vi "test_DL090211FPGA.vi"() -> ()   [LabVIEW 2010, in "FPGAWrapperDL090211Galvo.lvclass"]
uses:
  FPGAWrapperDL090211Galvo.lvclass
  common_typedefs/channels_cluster.ctl
  common_typedefs/gate_parameters_cluster.ctl
  common/classes/ErrorController/ErrorController/ErrorController.lvclass
  common/classes/ErrorController/ErrorController/class_data.vi
panel:
  in  "gate 1 settings":T1
  in  "channel offsets":T2
  out "error controller loaded?":bool=TRUE
  out "pixel dwell time":dbl[unit]
  out "timed out?":bool
  in  "timeout (ms)":i32=500
  out "DAQ loop counter":i32
  out "channel data block":dbl[][](graph)
  in  "number of channels":i32=3
  in  "block size":i32=10000
  out "DL090211FPGAWrapper out":refnum<class "FPGAWrapperDL090211Galvo.lvclass">
  in  "number of pixels":i64=1000000000
  in  "iterations per pixel":i32=250
  in  "run button":bool
  in  "stop":bool
  in  "create button":bool
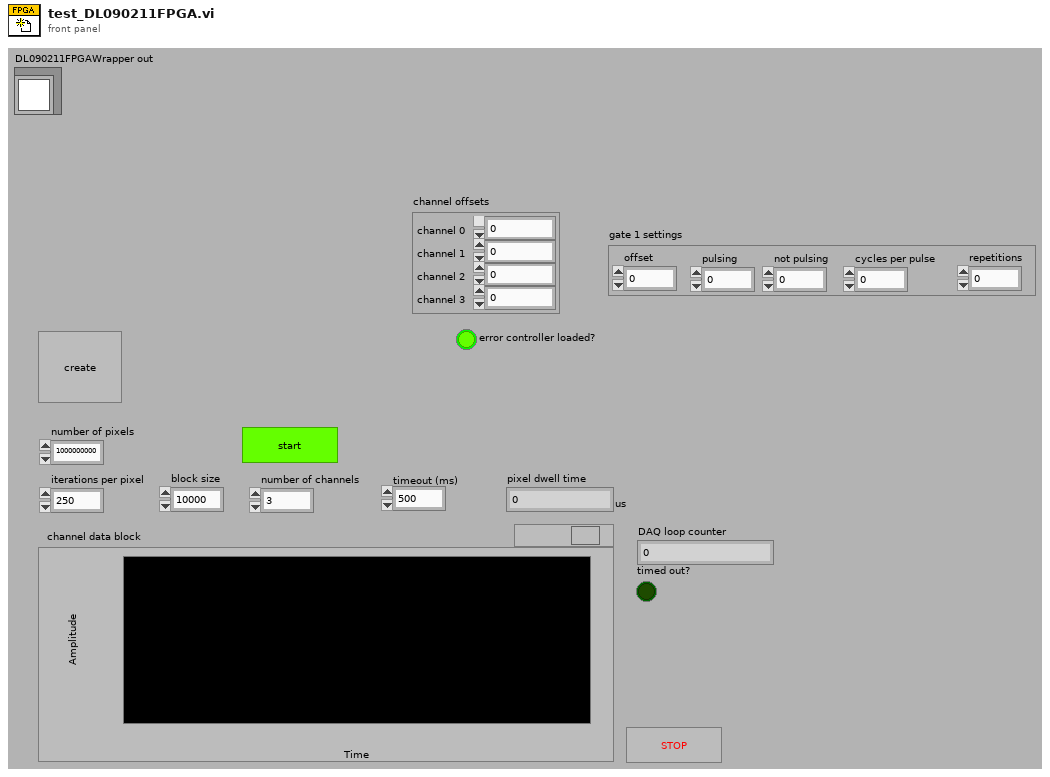
[diagram p1: front panel]
types:
  T1 = typedef "gate_parameters_cluster.ctl" = cluster{"offset":i64, "pulsing":i64, "not pulsing":i64, "cycles per pulse":i64, "repetitions":i64}
  T2 = typedef "channels_cluster.ctl" = cluster{"channel 0":u32, "channel 1":u32, "channel 2":u32, "channel 3":u32}
  T3 = typedef "pixel_raw_data_array.ctl" = dbl[][]
  T4 = typedef "plugin_specification.ctl" = cluster{"class path":string, "configuration":string, "label":string, "settings name":string}
  T5 = typedef "XComponentSpecification.xctl/data.ctl" = cluster{"class path":string, "configuration":string, "label":string, "settings name":string}
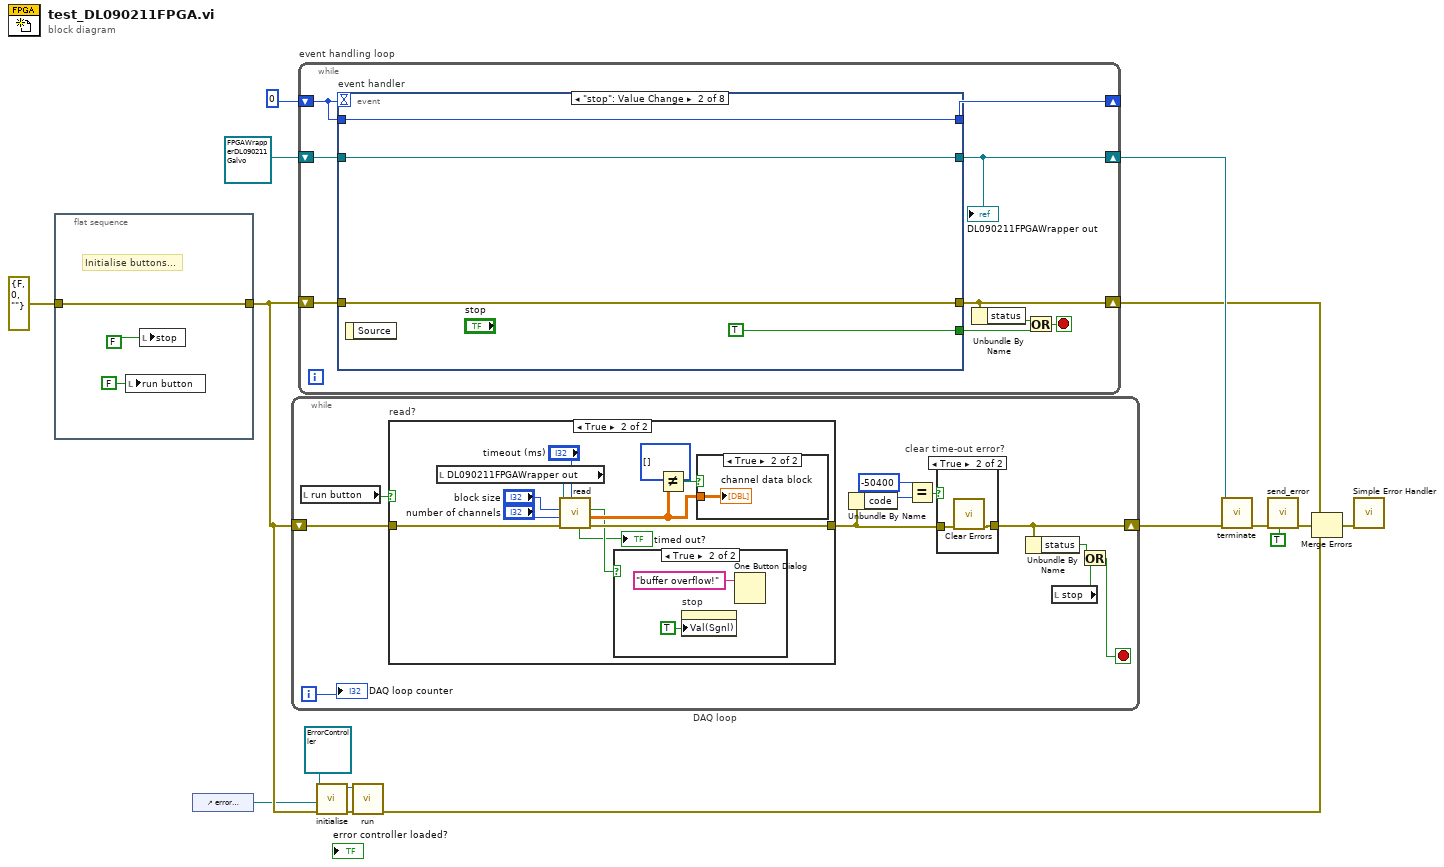
[diagram p0: block diagram]
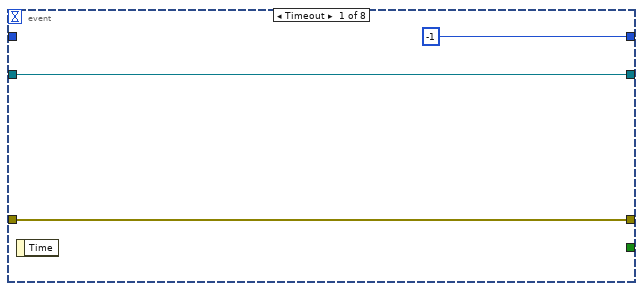
[diagram p6: hidden frame]
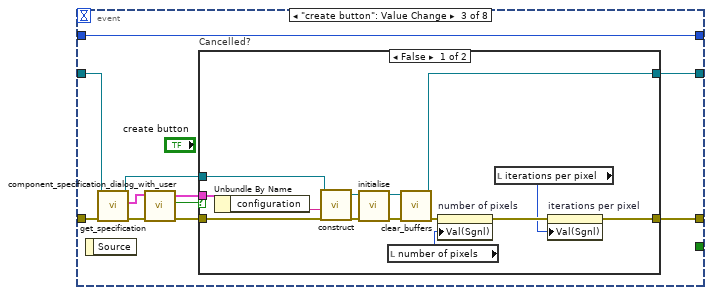
[diagram p7: hidden frame]
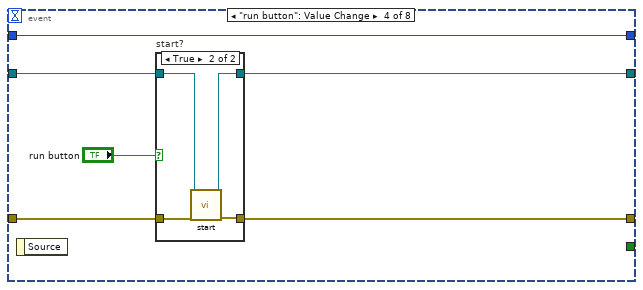
[diagram p9: hidden frame]
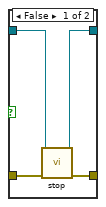
[diagram p10: hidden frame]
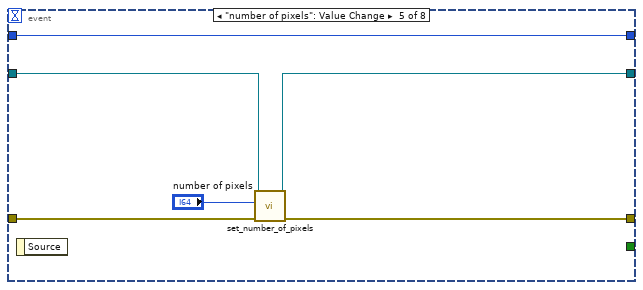
[diagram p11: hidden frame]
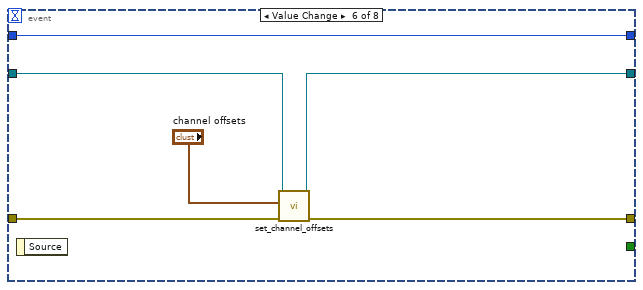
[diagram p12: hidden frame]
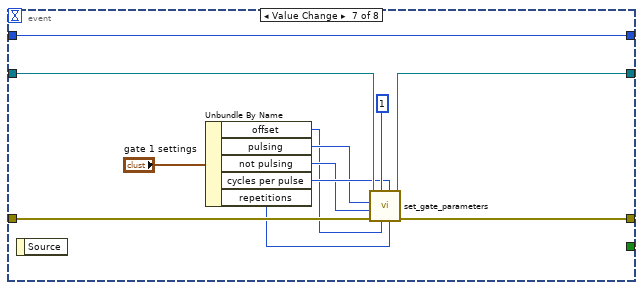
[diagram p13: hidden frame]
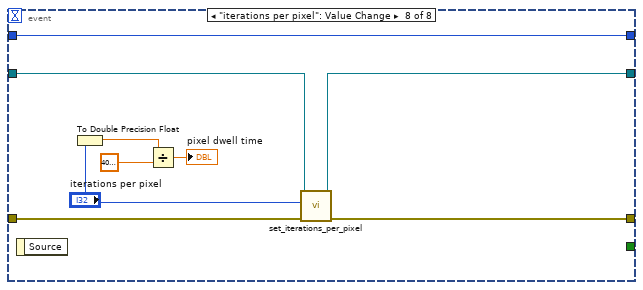
[diagram p14: hidden frame]
diagram:
  n1 = flat-sequence {
    tunnel: errorcluster {"status"=FALSE, "code"=0, "source"=""} ("error in (no error)") -> [w19]
    tunnel: [w19] -> w6
    frame #0 {
      # "Initialise buttons..."
      n2 = local write "run button"(FALSE ("run button")) -> ()
      n3 = local write "stop"(FALSE) -> ()
    }
  }
  n4 = control-ref of="error controller loaded?"() -> (w1:refnum<vi>)
  n5 = while "DAQ loop" {
    shift-right: [w24] -> w13
    shift-left: w6 -> [w30]
    i -> [w20]
    stop <- w21 stop-if-true
    n6 = local read "run button"() -> (w29:bool)
    n7 = case "read?" shown="True" w29 {
      tunnel: w30 -> [w34 w45]
      tunnel: [w34 w44] -> w26
      frame False {
      }
      frame True {
        n8 = local read "DL090211FPGAWrapper out"() -> (w43:refnum<class "FPGAWrapperDL090211Galvo.lvclass">)
        n9 = call-dynamic "read.vi"("timeout (ms)"="timeout (ms)", "error in (no error)"=w45, "number of channels"="number of channels", "block size"="block size", "FPGAWrapperDL090211Galvo in"=w43) -> ("error out"=w44:errorcluster, "channels raw data block"=w39:T3, "FIFO full?"=w37:bool, "timed out?"=→"timed out?":bool)  [unwired: 3 out]
        n10 = case shown="True" w37 {
          frame False {
          }
          frame True {
            n11 = property on="stop" class="Bool (strict)"("Val(Sgnl)"=TRUE) -> ()  [unwired: 2 in, 2 out]
            n12 = One Button Dialog(message="buffer overflow!") -> ()  [unwired: 1 in, 1 out]
          }
        }
        n13 = Not Equal?(x=i32[][] [], y=w39) -> (x != y?=w40:bool)
        n14 = case shown="True" w40 {
          tunnel: w39 -> [_ w48]
          frame False {
          }
          frame True {
            "channel data block" <- w48
          }
        }
      }
    }
    n15 = Unbundle By Name(w26) -> ("code"=w28:i32)
    n16 = Equal?(x=-50400, y=w28) -> (x = y?=w25:bool)
    n17 = case "clear time-out error?" shown="True" w25 {
      tunnel: w26 -> [w31 w33]
      tunnel: [w31 w32] -> w24
      frame False {
      }
      frame True {
        n18 = call <vilib>:"Clear Errors.vi"("error in (no error)"=w33) -> ("error out"=w32:errorcluster)  [unwired: 6 out]
      }
    }
    n19 = Unbundle By Name(w24) -> ("status"=w23:bool)
    n20 = local read "stop"() -> (w22:bool)
    n21 = Or(x=w23, y=w22) -> (x .or. y?=w21:bool)
    "DAQ loop counter" <- w20
  }
  n22 = while "event handling loop" {
    shift-right: [w52] -> w11
    shift-left: w6 -> [w57]
    shift-right: [w55] -> _
    shift-left: 0 -> [w56]
    shift-right: [w53] -> w12
    shift-left: refnum<class "FPGAWrapperDL090211Galvo.lvclass"> refnum ("DL090211FPGAWrapper.lvclass") -> [w54]
    stop <- w49 stop-if-true
    n23 = event "event handler" shown="[1] \"stop\": Value Change" {
      selector: _ -> [_ _ _ _ _ _ _ _]
      dyn-events: _ -> [_ _ _ _ _ _ _ _]
      timeout: w56 -> [_ _ _ _ _ _ _ _]
      tunnel: [w58 w61 w74 w93 w109 w115 w127 w136] -> w52
      tunnel: w57 -> [w58 w61 w71 w96 w110 w116 w128 w137]
      tunnel: w56 -> [_ w64 w75 w97 w111 w117 w129 w138]
      tunnel: [-1 w64 w75 w97 w111 w117 w129 w138] -> w55
      tunnel: [_ TRUE _ _ _ _ _ _] -> w50
      tunnel: [w59 w62 w66 w94 w107 w112 w125 w134] -> w53
      tunnel: w54 -> [w59 w62 w69 w95 w108 w113 w126 w135]
      event Timeout {
        n24 = event-data() -> ()  [unwired: 2 out]
      }
      event "stop": Value Change {
        n25 = event-data() -> ()  [unwired: 2 out]
      }
      event "create button": Value Change {
        n26 = event-data() -> ()  [unwired: 2 out]
        n27 = call-dynamic "get_specification.vi"("error in (no error)"=w71, "GenericPlugin in"=w69) -> ("error out"=w70:errorcluster, "component specification"=w67:T4, "GenericPlugin out"=w68:refnum<class "FPGAWrapperDL090211Galvo.lvclass">)  [unwired: 6 in, 1 out]
        n28 = call "component_specification_dialog_with_user.vi"("error in (no error)"=w70, "component specification in"=w67) -> ("error out"=w73:errorcluster, "cancelled?"=w65:bool, "component specification out"=w72:T5)  [unwired: 7 in]
        n29 = case "Cancelled?" shown="False" w65 {
          tunnel: [w86 w91] -> w74
          tunnel: w73 -> [w80 w91]
          tunnel: w72 -> [w79 _]
          tunnel: w68 -> [w77 w90]
          tunnel: [w76 w90] -> w66
          frame False {
            n30 = Unbundle By Name(w79) -> ("configuration"=w78:string)
            n31 = call-dynamic "construct.vi"("error in (no error)"=w80, "configuration name"=w78, "GenericPlugin in"=w77) -> ("error out"=w82:errorcluster, "GenericPlugin out"=w81:refnum<class "FPGAWrapperDL090211Galvo.lvclass">)  [unwired: 7 in]
            n32 = call-dynamic "initialise.vi"("error in (no error)"=w82, "GenericPlugin in"=w81) -> ("error out"=w85:errorcluster, "GenericPlugin out"=w83:refnum<class "FPGAWrapperDL090211Galvo.lvclass">)  [unwired: 1 in, 7 out]
            n33 = local read "number of pixels"() -> (w87:i64)
            n34 = call-dynamic "clear_buffers.vi"("error in (no error)"=w85, "FPGAWrapperDL090211Galvo in"=w83) -> ("error out"=w84:errorcluster, "FPGAWrapperDL090211Galvo out"=w76:refnum<class "FPGAWrapperDL090211Galvo.lvclass">)  [unwired: 8 in]
            n35 = property on="number of pixels" class="DigNum (strict)"(error in=w84, "Val(Sgnl)"=w87) -> (error out=w89:errorcluster)  [unwired: 1 in, 1 out]
            n36 = local read "iterations per pixel"() -> (w88:i32)
            n37 = property on="iterations per pixel" class="DigNum (strict)"(error in=w89, "Val(Sgnl)"=w88) -> (error out=w86:errorcluster)  [unwired: 1 in, 1 out]
          }
          frame True {
          }
        }
      }
      event "run button": Value Change {
        n38 = event-data() -> ()  [unwired: 2 out]
        n39 = case "start?" shown="True" "run button" {
          tunnel: w96 -> [w101 w105]
          tunnel: w95 -> [w99 w104]
          tunnel: [w98 w103] -> w94
          tunnel: [w100 w102] -> w93
          frame False {
            n40 = call-dynamic "stop.vi"("error in (no error)"=w101, "FPGAWrapperDL090211Galvo in"=w99) -> ("error out"=w100:errorcluster, "FPGAWrapperDL090211Galvo out"=w98:refnum<class "FPGAWrapperDL090211Galvo.lvclass">)  [unwired: 8 out]
          }
          frame True {
            n41 = call-dynamic "start.vi"("error in (no error)"=w105, "FPGAWrapperDL090211Galvo in"=w104) -> ("error out"=w102:errorcluster, "FPGAWrapperDL090211Galvo out"=w103:refnum<class "FPGAWrapperDL090211Galvo.lvclass">)  [unwired: 8 out]
          }
        }
      }
      event "number of pixels": Value Change {
        n42 = event-data() -> ()  [unwired: 2 out]
        n43 = call-dynamic "set_number_of_pixels.vi"("error in (no error)"=w110, "number of pixels"="number of pixels", "FPGAWrapperDL090211Galvo in"=w108) -> ("error out"=w109:errorcluster, "FPGAWrapperDL090211Galvo out"=w107:refnum<class "FPGAWrapperDL090211Galvo.lvclass">)  [unwired: 7 out]
      }
      event Value Change {
        n44 = event-data() -> ()  [unwired: 2 out]
        n45 = call-dynamic "set_channel_offsets.vi"("error in (no error)"=w116, "pixel values cluster"="channel offsets", "FPGAWrapperDL090211Galvo in"=w113) -> ("error out"=w115:errorcluster, "FPGAWrapperDL090211Galvo out"=w112:refnum<class "FPGAWrapperDL090211Galvo.lvclass">)  [unwired: 7 in]
      }
      event Value Change {
        n46 = event-data() -> ()  [unwired: 2 out]
        n47 = Unbundle By Name("gate 1 settings") -> ("offset"=w119:i64, "pulsing"=w121:i64, "not pulsing"=w120:i64, "cycles per pulse"=w122:i64, "repetitions"=w118:i64)
        n48 = call-dynamic "set_gate_parameters.vi"("repetitions"=w118, "pulse duration (iterations)"=w122, "offset duration (iterations)"=w119, "clock index"=1, "error in (no error)"=w128, "low phase duration (iterations)"=w120, "high phase duration (iterations)"=w121, "FPGAWrapperDL090211Galvo in"=w126) -> ("error out"=w127:errorcluster, "FPGAWrapperDL090211Galvo out"=w125:refnum<class "FPGAWrapperDL090211Galvo.lvclass">)  [unwired: 2 in]
      }
      event "iterations per pixel": Value Change {
        n49 = event-data() -> ()  [unwired: 2 out]
        n50 = To Double Precision Float(number="iterations per pixel") -> (double precision float=w132:dbl)
        n51 = Divide(x=w132, y=dbl[unit] 40000000.0) -> (x/y=→"pixel dwell time":dbl[unit])
        n52 = call-dynamic "set_iterations_per_pixel.vi"("error in (no error)"=w137, "iterations per pixel"="iterations per pixel", "FPGAWrapperDL090211Galvo in"=w135) -> ("error out"=w136:errorcluster, "FPGAWrapperDL090211Galvo out"=w134:refnum<class "FPGAWrapperDL090211Galvo.lvclass">)  [unwired: 7 out]
      }
    }
    "DL090211FPGAWrapper out" <- w53
    n53 = Unbundle By Name(w52) -> ("status"=w51:bool)
    n54 = Or(x=w51, y=w50) -> (x .or. y?=w49:bool)
  }
  n55 = call-dynamic "initialise.vi"("error in (no error)"=w6, "error boolean"=w1, "ErrorController in"=refnum<class "ErrorController.lvclass"> refnum) -> ("error out"=w9:errorcluster, "ErrorController out"=w8:refnum<class "ErrorController.lvclass">)  [unwired: 7 in]
  n56 = call "run.vi"("error in (no error)"=w9, "ErrorController in"=w8) -> ("error out"=w2:errorcluster)  [unwired: 8 in, 1 out]
  n57 = call-dynamic "terminate.vi"("error in (no error)"=w13, "GenericPlugin in"=w12) -> ("error out"=w5:errorcluster)  [unwired: 9 out]
  n58 = call "send_error.vi"("last error? (F)"=TRUE, "error in (no error)"=w5) -> ("error out"=w4:errorcluster)  [unwired: 9 in]
  n59 = Merge Errors(w11, w4, w2) -> (w10:errorcluster)
  n60 = call <vilib>:"Simple Error Handler.vi"("error in (no error)"=w10) -> ()  [unwired: 1 in, 8 out]
